vi "Z_Q_5000.vi"(9 "Type":string) -> (0 "Qn":dbl[](array[numeric]), 2 "L":i32)   [LabVIEW 2019]
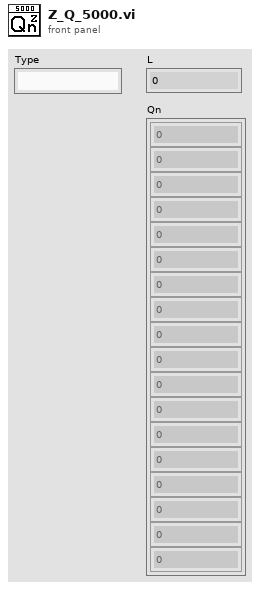
[diagram p1: front panel]
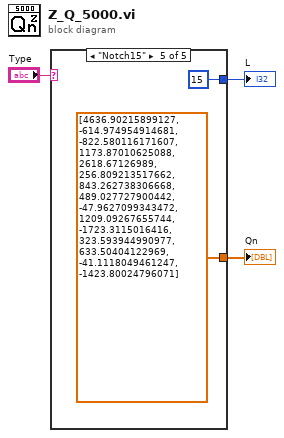
[diagram p0: block diagram]
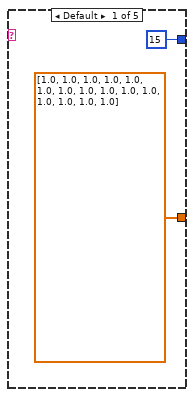
[diagram p2: hidden frame]
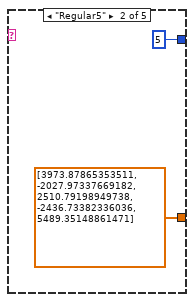
[diagram p3: hidden frame]
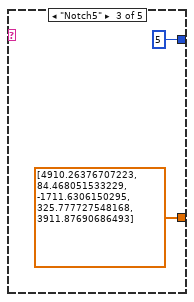
[diagram p4: hidden frame]
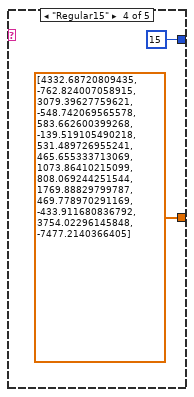
[diagram p5: hidden frame]
diagram:
  n1 = case shown="\"Notch15\"" "Type" {
    tunnel: [15 5 5 15 15] -> w2
    tunnel: [dbl[] [1.0, 1.0, 1.0, 1.0, 1.0, 1.0, 1.0, 1.0, 1.0, 1.0, 1.0, 1.0, 1.0, 1.0, 1.0] ("Qn") dbl[] [3973.87865353511, -2027.97337669182, 2510.79198949738, -2436.73382336036, 5489.35148861471] ("Qn") dbl[] [4910.26376707223, 84.468051533229, -1711.6306150295, 325.777727548168, 3911.87690686493] ("Qn") dbl[] [4332.68720809435, -762.824007058915, 3079.39627759621, -548.742069565578, 583.662600399268, -139.519105490218, 531.489726955241, 465.655333713069, 1073.86410215099, 808.069244251544, 1769.88829799787, 469.778970291169, -433.911680836792, 3754.02296145848, -7477.2140366405] ("Qn") dbl[] [4636.90215899127, -614.974954914681, -822.580116171607, 1173.87010625088, 2618.67126989, 256.809213517662, 843.262738306668, 489.027727900442, -47.9627099343472, 1209.09267655744, -1723.3115016416, 323.593944990977, 633.50404122969, -41.1118049461247, -1423.80024796071] ("Qn")] -> w1
    frame Default {
    }
    frame "Regular5" {
    }
    frame "Notch5" {
    }
    frame "Regular15" {
    }
    frame "Notch15" {
    }
  }
  "Qn" <- w1
  "L" <- w2
